vi "Heat Up Macro Find Step.vi"(8 "Error In":errorcluster, 10 "Search For Step Name":string, 11 "Heat Up Data with Only Selected Columns":string[][](array[string])) -> (0 "Error Out":errorcluster, 2 "Index":i32[](array[numeric]), 3 "Filtered Array":string[][](array[string]))   [LabVIEW 2019]
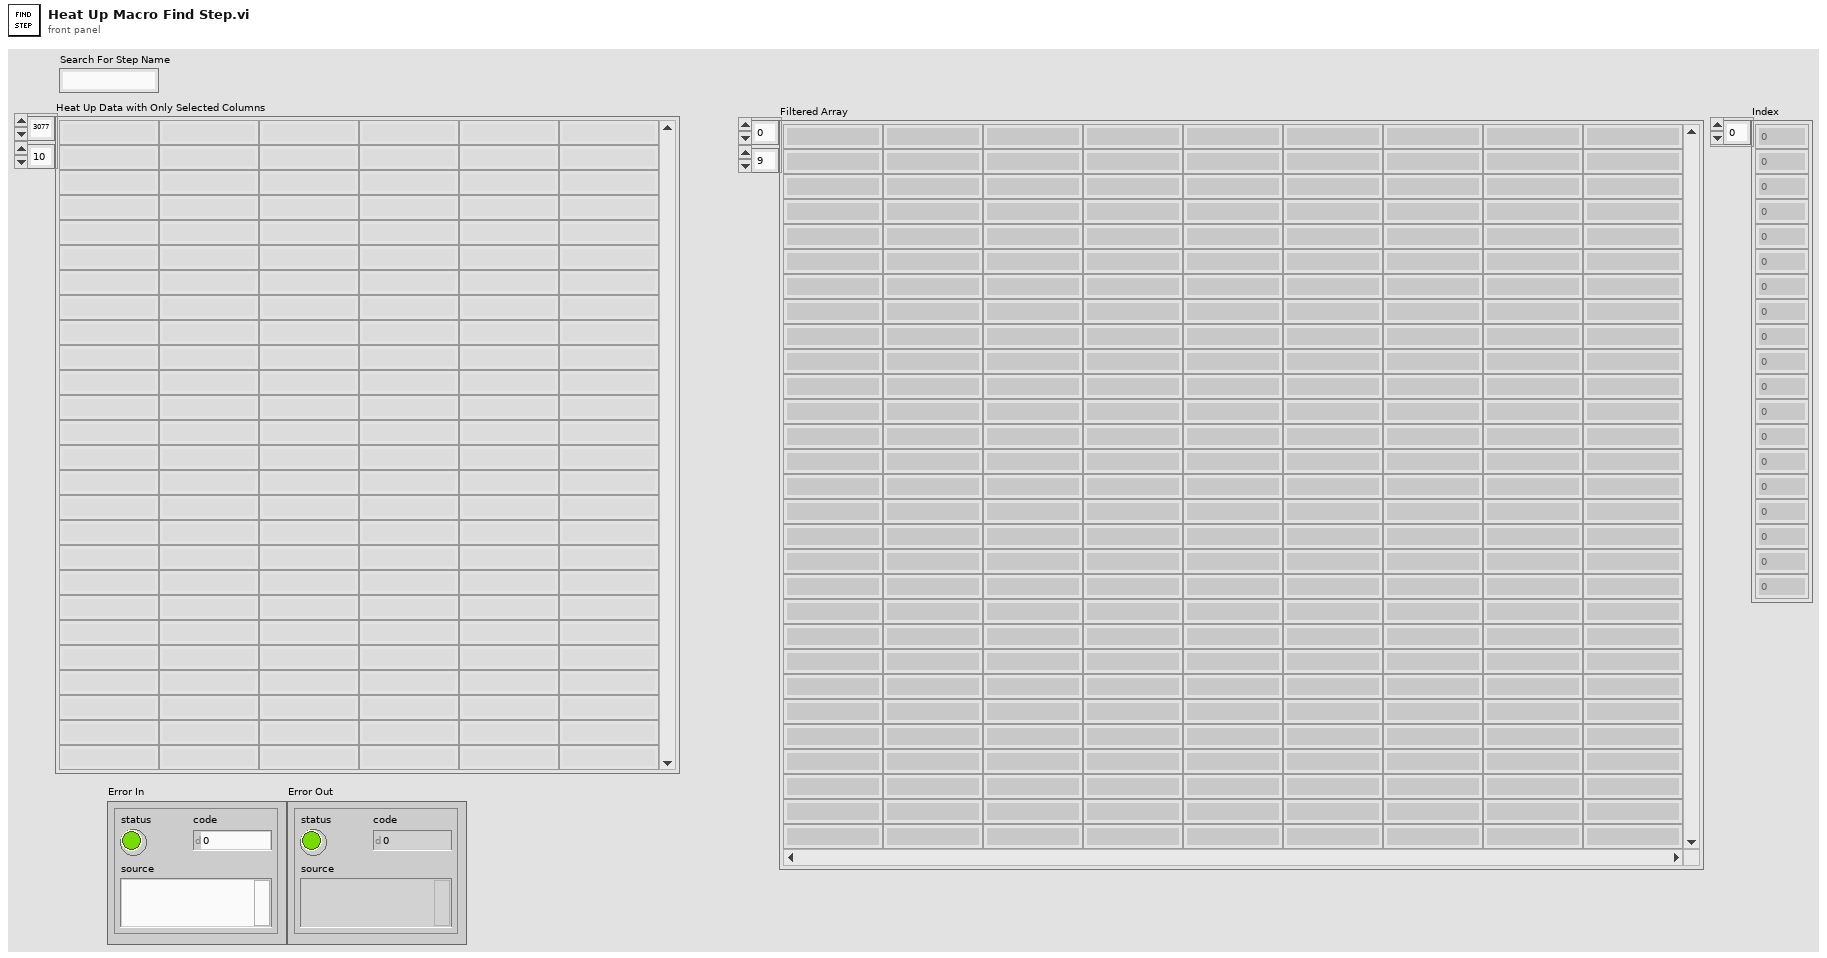
[diagram p1: front panel]
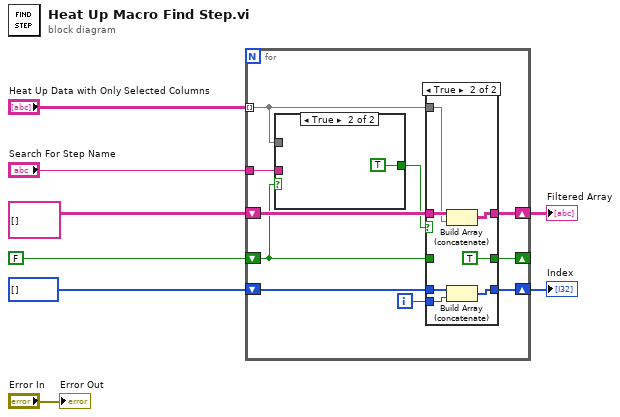
[diagram p0: block diagram]
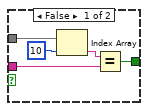
[diagram p2: hidden frame]
diagram:
  n1 = for {
    tunnel: "Heat Up Data with Only Selected Columns" -> [w16] mode=indexing
    shift-right: [w17] -> w6
    shift-left: string[][] [] -> [w18]
    shift-right: [w13] -> _
    shift-left: FALSE -> [w14]
    shift-right: [w11] -> w2
    shift-left: i32[] [] -> [w12]
    tunnel: "Search For Step Name" -> [w9]
    i -> [w10]
    n2 = case shown="True" w14 {
      tunnel: w16 -> [w21 _]
      tunnel: [w20 TRUE] -> w15
      tunnel: w9 -> [w19 _]
      frame False {
        n3 = Index Array(array=w21, index=10 ("disabled index (col)")) -> (element=w23:string)
        n4 = Equal?(x=w23, y=w19) -> (x = y?=w20:bool)
      }
      frame True {
      }
    }
    n5 = case shown="True" w15 {
      tunnel: w18 -> [w27 w34]
      tunnel: [w27 w33] -> w17
      tunnel: w16 -> [_ w32]
      tunnel: [w26 TRUE] -> w13
      tunnel: w14 -> [w26 _]
      tunnel: w12 -> [w25 w30]
      tunnel: [w25 w29] -> w11
      tunnel: w10 -> [_ w28]
      frame False {
      }
      frame True {
        n6 = Build Array (concatenate)(w34, w32) -> (w33:string[][])
        n7 = Build Array (concatenate)(w30, w28) -> (w29:i32[])
      }
    }
  }
  "Filtered Array" <- w6
  "Index" <- w2
  "Error Out" <- "Error In"
